vi "CreateSelfReference.vi"(8 "error in (no error)":errorcluster, 11 "SMO":refnum<class "SMO.Template.lvclass">) -> (0 "error out":errorcluster, 3 "SMO out":refnum<class "SMO.Template.lvclass">)   [LabVIEW 2013, in "SMO.Template.lvclass"]
uses:
  SMO.Template.lvclass
  SMO/SMO.lvclass
  SMO.Template.lvclass/SMO.Template.ctl
panel:
  # "For instructions on how to use the JKI State Machine Objects, examples and video tutorials, visit:\nhttp://jki.net/state-machine-objects/\n\nJKI State Machine Objects™\nhttp://jki.net/state-machine-objects/\nCopyright (C) 2005-2015, JKI <info@jki.net>\nALL RIGHTS RESERVED"
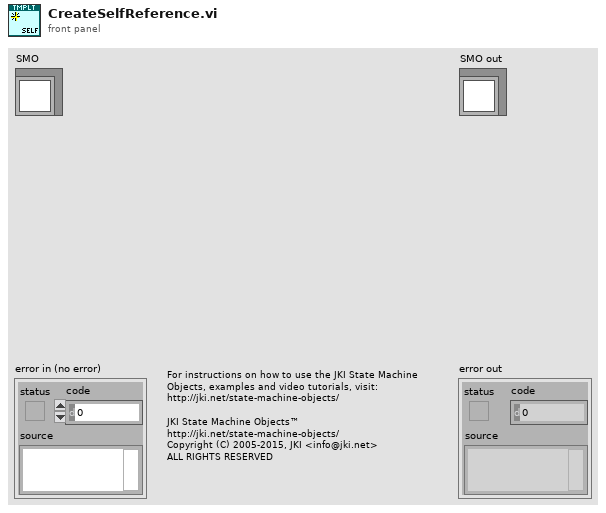
[diagram p1: front panel]
types:
  T1 = typedef "SMO.Template.lvclass/PrivateData--Ref.ctl" = refnum<data-value>
  T2 = typedef "SMO.Template.lvclass/PrivateData--Cluster.ctl" = cluster{"Configuration":T3, "Public Events":T4, "Protected Events":T5, "Data":string}
  T3 = typedef "SMO.Template.lvclass/Configuration--Cluster.ctl" = cluster{"Suffix":string}
  T4 = typedef "SMO.Template.lvclass/PublicEvents--Cluster.ctl" = cluster{"Data Changed":refnum<user-event>}
  T5 = typedef "SMO.Template.lvclass/ProtectedEvents--Cluster.ctl" = cluster{"API_Template":refnum<user-event>}
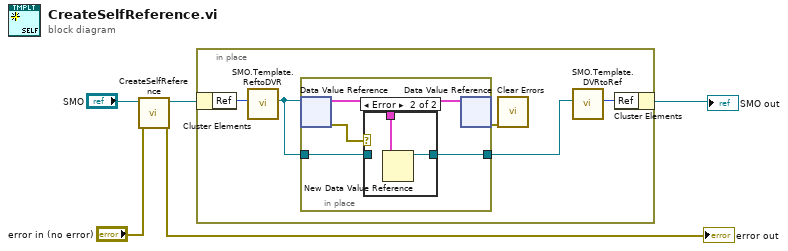
[diagram p0: block diagram]
diagram:
  n1 = call-parent "CreateSelfReference.vi"("error in (no error)"="error in (no error)", "SMO"="SMO") -> ("error out"=→"error out":errorcluster, "SMO out"=w4:refnum<class "SMO.Template.lvclass">)  [unwired: 8 in]
  n2 = in-place {
    n3 = in-place-cluster #1(w4) -> ("Ref"=w10:u32)
    n4 = call "SMO.Template.ReftoDVR.vi"("Ref"=w10) -> ("Ref"=w9:T1)  [unwired: 10 in]
    n5 = in-place {
      in-place-border: [w14] -> w7
      in-place-border: w9 -> [w11]
      n6 = in-place-dvr #2(w9) -> (w13:T2, w12:errorcluster)
      n7 = case shown="Error" w12 {
        tunnel: [w15 w17] -> w14
        tunnel: w13 -> [_ w16]
        tunnel: w11 -> [w15 _]
        frame No Error {
        }
        frame Error {
          n8 = New Data Value Reference(data value=w16) -> (data value reference=w17:refnum<data-value>)  [unwired: 1 in, 1 out]
        }
      }
      n9 = in-place-dvr #2(w13) -> (w6:errorcluster)  [unwired: 1 out]
    }
    n10 = call <vilib>:"Clear Errors.vi"("error in (no error)"=w6) -> ()  [unwired: 6 in, 1 out]
    n11 = call "SMO.Template.DVRtoRef.vi"("Ref"=w7) -> ("Ref"=w8:u32)  [unwired: 10 in]
    n12 = in-place-cluster #1("Ref"=w8) -> (→"SMO out":refnum<class "SMO.Template.lvclass">)
  }
